vi "String2UTF8.vi"(10 "error in":errorcluster, 11 "text":string) -> (2 "error out":errorcluster, 3 "utf-8 text":string)   [LabVIEW 2020, in "Common.lvlib"]
uses:
  Common.lvlib
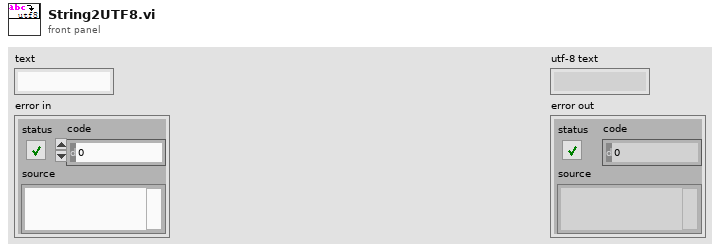
[diagram p1: front panel]
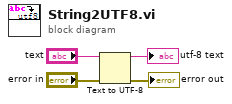
[diagram p0: block diagram]
diagram:
  n1 = Text to UTF-8(8:"error in", 11:"text") -> (0:→"error out":errorcluster, 3:→"utf-8 text":string)  [unwired: 1 in]
